vi "Create All Message Queues.vi"(8 "error in (no error)":errorcluster) -> (0 "error out":errorcluster, 3 "Message Queues out":T1)   [LabVIEW 2025, in "LAB-IQ Message Queue.lvlib"]
doc: "This VI creates and initializes all the message queues for your application. If your application requires more than one message queue, right-click the \"Message Queues\" constant above and select Open Type Def. Add the new Message Queue(s) to the type definition, then initialize them in this VI."
uses:
  LAB-IQ Message Queue.lvlib
  All Message Queues.ctl
  Message Cluster.ctl
  Enqueue Message (Single).vi
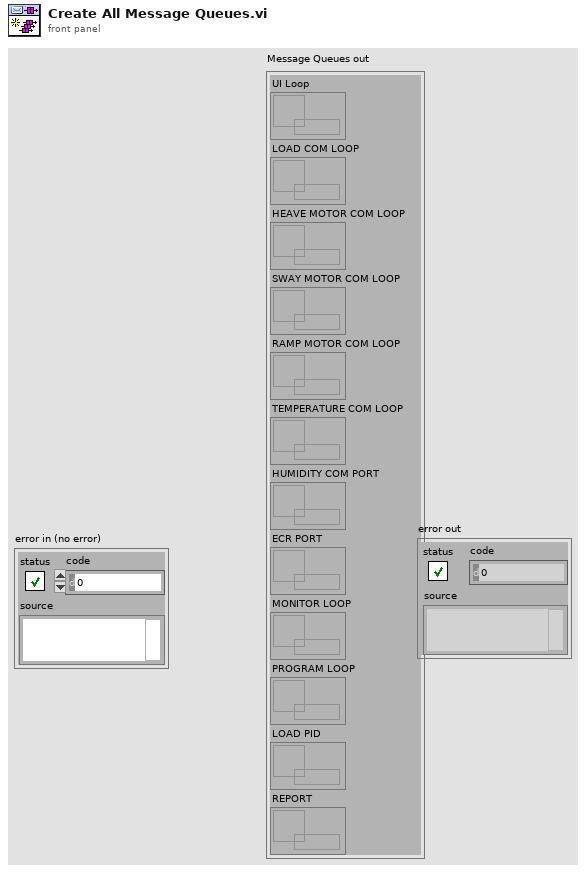
[diagram p1: front panel]
types:
  T1 = typedef "LAB-IQ Message Queue.lvlib/All Message Queues.ctl" = cluster{"UI Loop":refnum<queue>, "LOAD COM LOOP":refnum<queue>, "HEAVE MOTOR COM LOOP":refnum<queue>, "SWAY MOTOR COM LOOP":refnum<queue>, "RAMP MOTOR COM LOOP":refnum<queue>, "TEMPERATURE COM LOOP":refnum<queue>, "HUMIDITY COM PORT":refnum<queue>, "ECR PORT":refnum<queue>, "MONITOR LOOP":refnum<queue>, "PROGRAM LOOP":refnum<queue>, "LOAD PID":refnum<queue>, "REPORT":refnum<queue>}
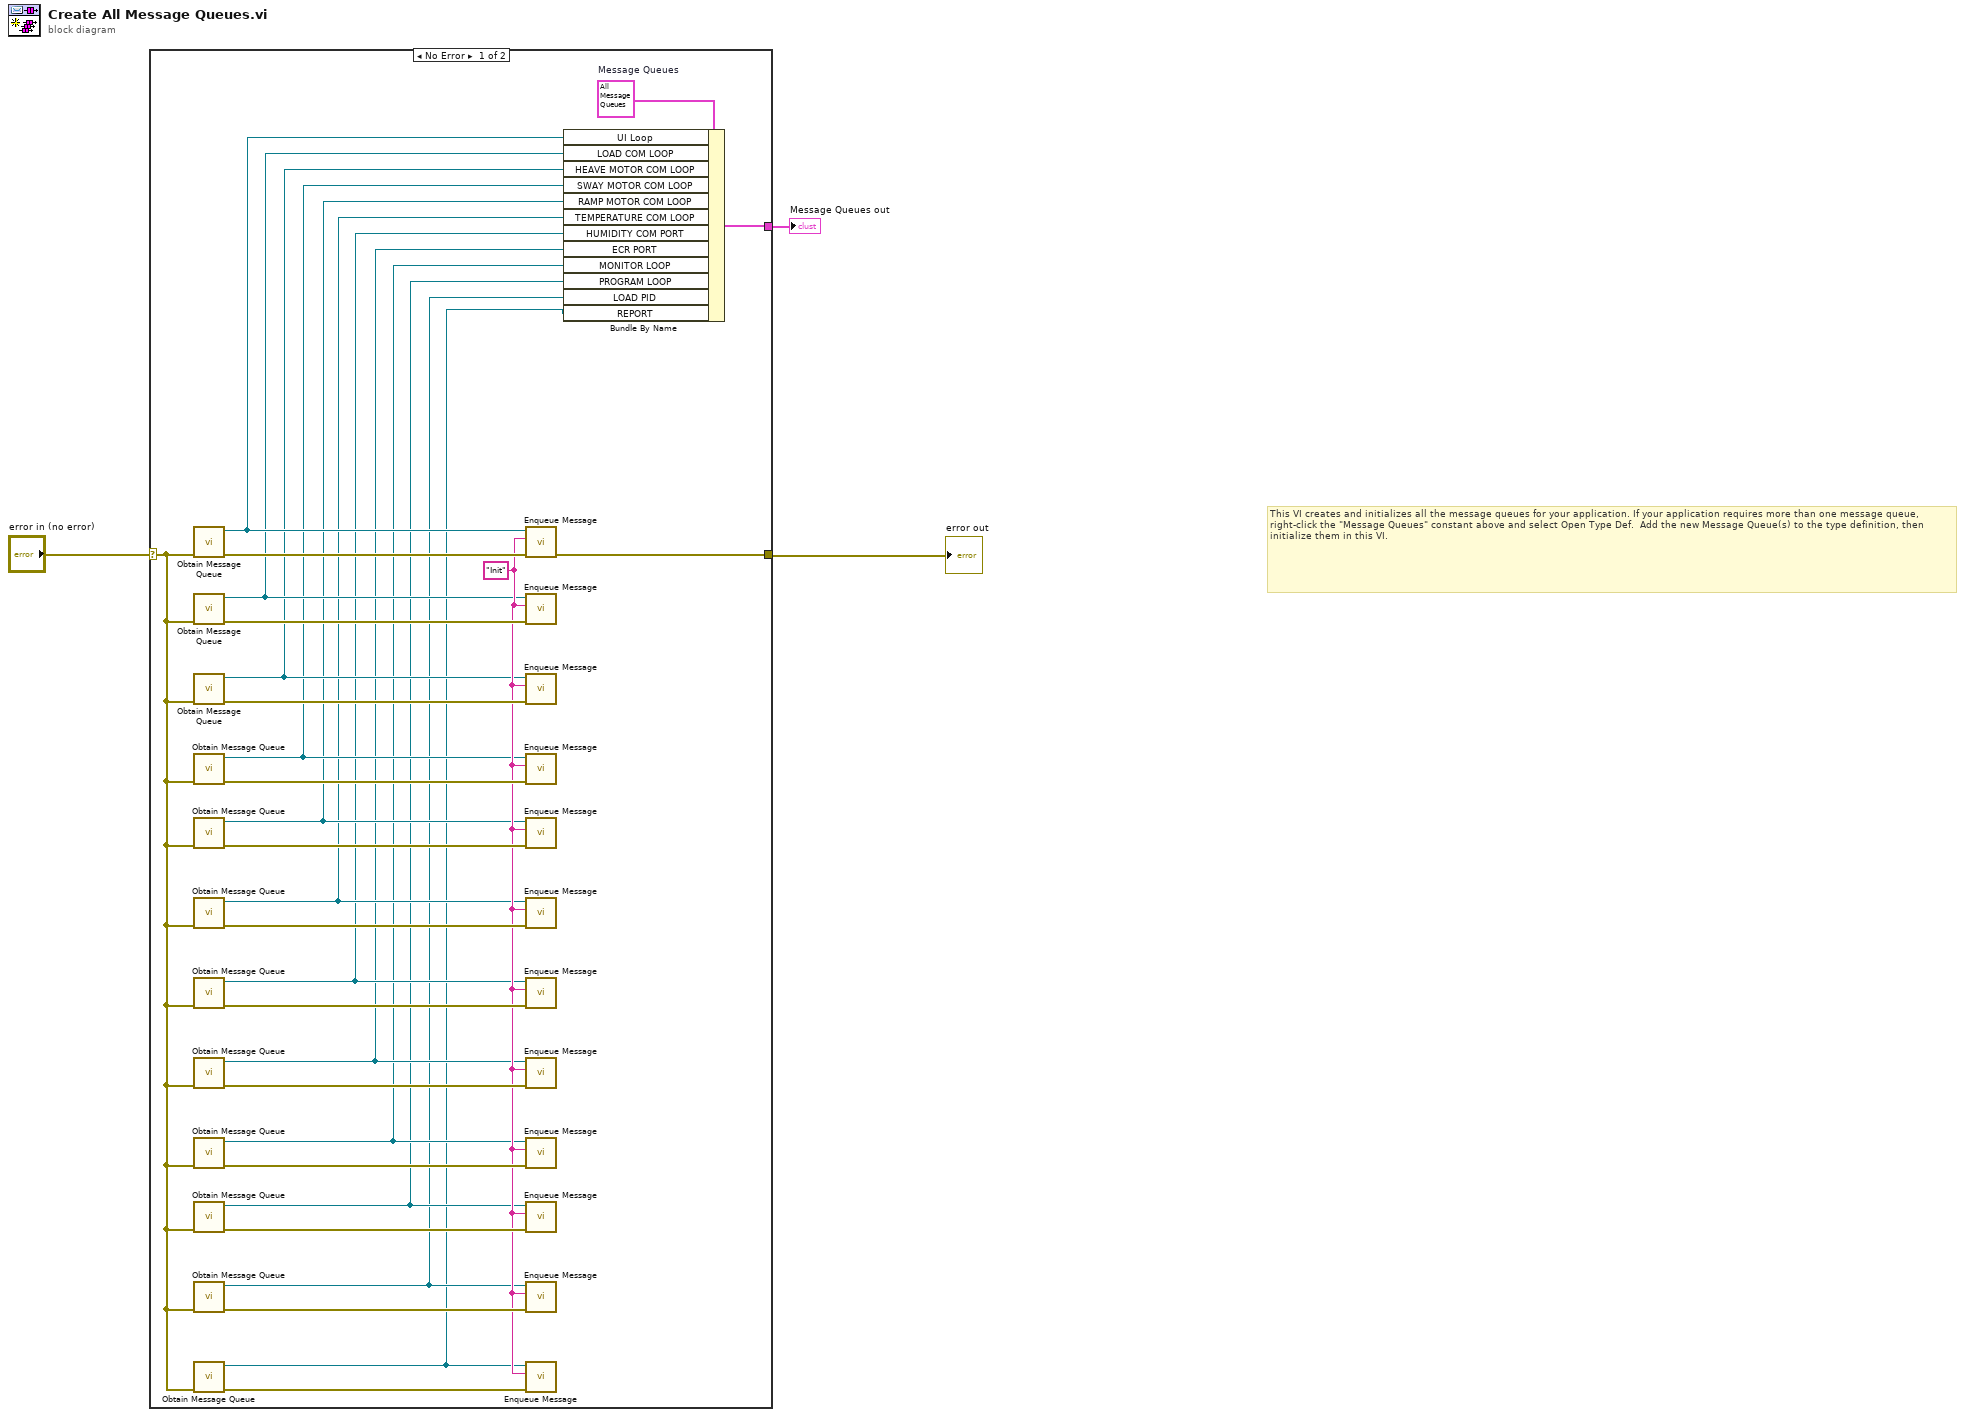
[diagram p0: block diagram]
diagram:
  # "This VI creates and initializes all the message queues for your application. If your application requires more than one message queue, right-click the \"Message Queues\" constant above and select Open Type Def.  Add the new Message Queue(s) to the type definition, then initialize them in this VI."
  n1 = case shown="No Error" "error in (no error)" {
    selector: "error in (no error)" -> [w16 w33]
    tunnel: [w32 w33] -> w3
    tunnel: [w30 _] -> w2
    frame No Error {
      w15 = "Init" ("Message")
      w31 = T1 {"UI Loop"=refnum, "LOAD COM LOOP"=refnum, "HEAVE MOTOR COM LOOP"=refnum, "SWAY MOTOR COM LOOP"=refnum, "RAMP MOTOR COM LOOP"=refnum, "TEMPERATURE COM LOOP"=refnum, "HUMIDITY COM PORT"=refnum, "ECR PORT"=refnum, "MONITOR LOOP"=refnum, "PROGRAM LOOP"=refnum, "LOAD PID"=refnum, "REPORT"=refnum}  # Message Queues
      n2 = call "Obtain Message Queue.vi"("error in (no error)"=w16) -> ("error out"=w29:errorcluster, "Message Queue"=w28:refnum<queue>)  [unwired: 9 in]
      n3 = call "Obtain Message Queue.vi"("error in (no error)"=w16) -> ("error out"=w27:errorcluster, "Message Queue"=w14:refnum<queue>)  [unwired: 9 in]
      n4 = call "Obtain Message Queue.vi"("error in (no error)"=w16) -> ("error out"=w26:errorcluster, "Message Queue"=w13:refnum<queue>)  [unwired: 9 in]
      n5 = call "Obtain Message Queue.vi"("error in (no error)"=w16) -> ("error out"=w25:errorcluster, "Message Queue"=w12:refnum<queue>)  [unwired: 9 in]
      n6 = call "Obtain Message Queue.vi"("error in (no error)"=w16) -> ("error out"=w22:errorcluster, "Message Queue"=w11:refnum<queue>)  [unwired: 9 in]
      n7 = call "Obtain Message Queue.vi"("error in (no error)"=w16) -> ("error out"=w23:errorcluster, "Message Queue"=w10:refnum<queue>)  [unwired: 9 in]
      n8 = call "Obtain Message Queue.vi"("error in (no error)"=w16) -> ("error out"=w24:errorcluster, "Message Queue"=w9:refnum<queue>)  [unwired: 9 in]
      n9 = call "Obtain Message Queue.vi"("error in (no error)"=w16) -> ("error out"=w17:errorcluster, "Message Queue"=w8:refnum<queue>)  [unwired: 9 in]
      n10 = call "Obtain Message Queue.vi"("error in (no error)"=w16) -> ("error out"=w18:errorcluster, "Message Queue"=w7:refnum<queue>)  [unwired: 9 in]
      n11 = call "Obtain Message Queue.vi"("error in (no error)"=w16) -> ("error out"=w21:errorcluster, "Message Queue"=w6:refnum<queue>)  [unwired: 9 in]
      n12 = call "Obtain Message Queue.vi"("error in (no error)"=w16) -> ("error out"=w20:errorcluster, "Message Queue"=w5:refnum<queue>)  [unwired: 9 in]
      n13 = call "Obtain Message Queue.vi"("error in (no error)"=w16) -> ("error out"=w19:errorcluster, "Message Queue"=w4:refnum<queue>)  [unwired: 9 in]
      n14 = call-poly "Enqueue Message.vi"("error in (no error)"=w29, "Message"=w15, "Message Queue"=w28) -> ("error out"=w32:errorcluster)  [unwired: 7 in, 1 out]
      n15 = call-poly "Enqueue Message.vi"("error in (no error)"=w27, "Message"=w15, "Message Queue"=w14) -> ()  [unwired: 7 in, 2 out]
      n16 = call-poly "Enqueue Message.vi"("error in (no error)"=w26, "Message"=w15, "Message Queue"=w13) -> ()  [unwired: 7 in, 2 out]
      n17 = call-poly "Enqueue Message.vi"("error in (no error)"=w25, "Message"=w15, "Message Queue"=w12) -> ()  [unwired: 7 in, 2 out]
      n18 = call-poly "Enqueue Message.vi"("error in (no error)"=w22, "Message"=w15, "Message Queue"=w11) -> ()  [unwired: 7 in, 2 out]
      n19 = call-poly "Enqueue Message.vi"("error in (no error)"=w23, "Message"=w15, "Message Queue"=w10) -> ()  [unwired: 7 in, 2 out]
      n20 = call-poly "Enqueue Message.vi"("error in (no error)"=w24, "Message"=w15, "Message Queue"=w9) -> ()  [unwired: 7 in, 2 out]
      n21 = call-poly "Enqueue Message.vi"("error in (no error)"=w17, "Message"=w15, "Message Queue"=w8) -> ()  [unwired: 7 in, 2 out]
      n22 = call-poly "Enqueue Message.vi"("error in (no error)"=w18, "Message"=w15, "Message Queue"=w7) -> ()  [unwired: 7 in, 2 out]
      n23 = call-poly "Enqueue Message.vi"("error in (no error)"=w21, "Message"=w15, "Message Queue"=w6) -> ()  [unwired: 7 in, 2 out]
      n24 = call-poly "Enqueue Message.vi"("error in (no error)"=w20, "Message"=w15, "Message Queue"=w5) -> ()  [unwired: 7 in, 2 out]
      n25 = call-poly "Enqueue Message.vi"("error in (no error)"=w19, "Message"=w15, "Message Queue"=w4) -> ()  [unwired: 7 in, 2 out]
      n26 = Bundle By Name(cluster=w31, "UI Loop"=w28, "LOAD COM LOOP"=w14, "HEAVE MOTOR COM LOOP"=w13, "SWAY MOTOR COM LOOP"=w12, "RAMP MOTOR COM LOOP"=w11, "TEMPERATURE COM LOOP"=w10, "HUMIDITY COM PORT"=w9, "ECR PORT"=w8, "MONITOR LOOP"=w7, "PROGRAM LOOP"=w6, "LOAD PID"=w5, "REPORT"=w4) -> (w30:T1)
    }
    frame Error {
    }
  }
  "Message Queues out" <- w2
  "error out" <- w3
